vi "Custom saving path GUI.vi"(8 "error in (no error)":errorcluster, 11 "DAQOrcaFlash in":refnum<class "DAQOrcaFlash.lvclass">) -> (0 "error out":errorcluster, 3 "DAQOrcaFlash out":refnum<class "DAQOrcaFlash.lvclass">)   [LabVIEW 2012, in "DAQOrcaFlash.lvclass"]
uses:
  DAQOrcaFlash.lvclass
  <vilib>/Distrio/Murmex/Murmex/Murmex.lvclass
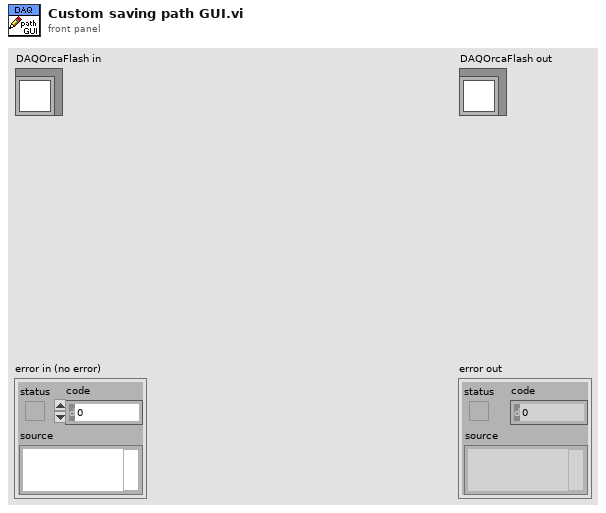
[diagram p1: front panel]
types:
  T1 = enum8{"Enabled", "Disabled", "Disabled and Grayed Out"}
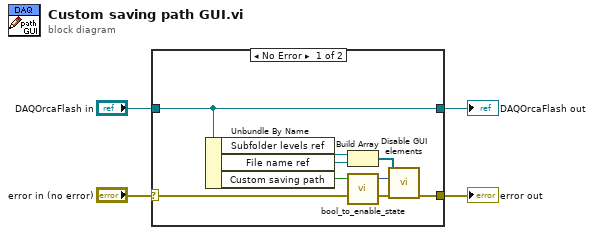
[diagram p0: block diagram]
diagram:
  n1 = case shown="No Error" "error in (no error)" {
    selector: "error in (no error)" -> [w11 w14]
    tunnel: [w10 w14] -> w3
    tunnel: [w12 w13] -> w1
    tunnel: "DAQOrcaFlash in" -> [w12 w13]
    frame No Error {
      n2 = Unbundle By Name(w12) -> ("Subfolder levels ref"=w9:refnum<vi>, "File name ref"=w8:refnum<vi>, "Custom saving path"=w5:bool)
      n3 = Build Array(w9, w8) -> (w7:refnum<vi>[])
      n4 = call "bool_to_enable_state.vi"("boolean in"=w5) -> ("enabled status out"=w6:T1)  [unwired: 4 in]
      n5 = call <vilib>:"Disable GUI elements.vi"("error in (no error)"=w11, "enabled state"=w6, "control refs"=w7) -> ("error out"=w10:errorcluster)  [unwired: 8 in]
    }
    frame Error {
    }
  }
  "error out" <- w3
  "DAQOrcaFlash out" <- w1
